vi "Set DO.vi"(0 "Module Ref":refnum<class "Modbus Master.lvclass">, 5 "Channel 0":bool, 7 "Channel 1":bool, 11 "error in (no error)":errorcluster) -> (4 "Modbus master out":refnum<class "Modbus Master.lvclass">, 15 "error out":errorcluster)   [LabVIEW 2024]
doc: "Set digital output states."
uses:
  <vilib>/NI/Modbus Library/API/Master/Modbus Master.lvclass
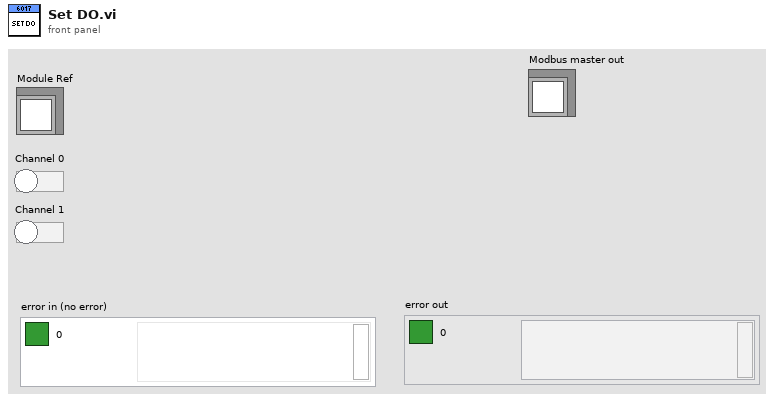
[diagram p1: front panel]
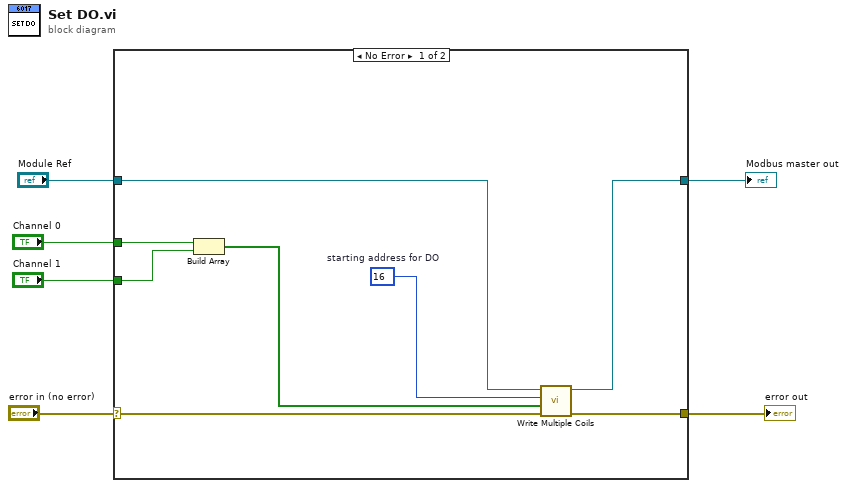
[diagram p0: block diagram]
diagram:
  n1 = case shown="No Error" "error in (no error)" {
    selector: "error in (no error)" -> [w14 w15]
    tunnel: "Module Ref" -> [w11 w16]
    tunnel: [w13 w15] -> w4
    tunnel: [w10 w16] -> w3
    tunnel: "Channel 0" -> [w9 _]
    tunnel: "Channel 1" -> [w8 _]
    frame No Error {
      w12 = u16 16  # starting address for DO
      n2 = Build Array(w9, w8) -> (w7:bool[])
      n3 = call-dynamic "Write Multiple Coils.vi"("error in"=w14, "coils to write"=w7, "starting address"=w12, "Modbus master in"=w11) -> ("error out"=w13:errorcluster, "Modbus master out"=w10:refnum<class "Modbus Master.lvclass">)  [unwired: 6 in]
    }
    frame Error {
    }
  }
  "error out" <- w4
  "Modbus master out" <- w3
